vi "Launcher.vi"   [LabVIEW 2020]
uses:
  Controllers/UI Controller/UI Controller/UI Controller.lvclass
  C:/Program Files/National Instruments/LabVIEW 2020/vi.lib/ActorFramework/Actor/Actor.lvclass
  Controllers/UI Controller/Factories/Full Factory/Full Factory.lvclass
  E:/Git/Labview-Projects/Completed projects/Map Editor/Controllers/UI Controller/Factories/UI Factory/UI Factory.lvclass
  Controllers/UI Controller/UI Controller/UI Controller.lvclass/UI Controller.ctl
  <vilib>/ActorFramework/Actor/Actor.lvclass
panel:
  # "NOTICE -- YOU MUST LEAVE THIS NOTICE IN PLACE.\n\nCopyright (c) 2017, LIANG LIU Shawn.Liu.cn@gmail.com\nAll rights reserved.\n\nRedistribution and use in source and binary forms, with or without modification, are permitted provided that the following conditions are met:\n-Redistributions of source code must retain the above copyright notice, this list of conditions and the following disclaimer.\n-Redistributions in binary form must reproduce the above copyright notice, this list of conditions and the following disclaimer in the documentation and/or other materials provided with the distribution.\n-Neither the name of the eLp nor the names of its contributors may be used to endorse or promote products derived from this software without specific prior written permission.\n\nTHIS SOFTWARE IS PROVIDED BY THE COPYRIGHT HOLDERS AND CONTRIBUTORS \"AS IS\" AND ANY EXPRESS OR IMPLIED WARRANTIES, INCLUDING, BUT NOT LIMITED TO, THE IMPLIED WARRANTIES OF MERCHANTABILITY AND FITNESS FOR A PARTICULAR PURPOSE ARE DISCLAIMED. IN NO EVENT SHALL THE COPYRIGHT HOLDER OR CONTRIBUTORS BE LIABLE FOR ANY DIRECT, INDIRECT, INCIDENTAL, SPECIAL, EXEMPLARY, OR CONSEQUENTIAL DAMAGES (INCLUDING, BUT NOT LIMITED TO, PROCUREMENT OF SUBSTITUTE GOODS OR SERVICES; LOSS OF USE, DATA, OR PROFITS; OR BUSINESS INTERRUPTION) HOWEVER CAUSED AND ON ANY THEORY OF LIABILITY, WHETHER IN CONTRACT, STRICT LIABILITY, OR TORT (INCLUDING NEGLIGENCE OR OTHERWISE) ARISING IN ANY WAY OUT OF THE USE OF THIS SOFTWARE, EVEN IF ADVISED OF THE POSSIBILITY OF SUCH DAMAGE."
types:
  T1 = enum32{"invalid app kind", "Development System", "Run Time System", "Student Edition", "Embedded LabVIEW", "Evaluation", "Custom"}
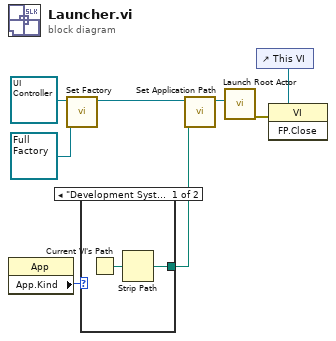
[diagram p0: block diagram]
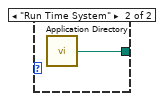
[diagram p2: hidden frame]
diagram:
  n1 = property class="App"() -> ("App.Kind"=w2:T1)  [unwired: 2 in, 2 out]
  n2 = call "Set Factory.vi"("Factory"=refnum<class "Full Factory.lvclass"> refnum ("UI Controller.lvlib:Full Factory.lvclass"), "UI Controller in"=refnum<class "UI Controller.lvclass"> refnum ("UI Controller.lvlib:UI Controller.lvclass")) -> ("UI Controller out"=w7:refnum<class "UI Controller.lvclass">)  [unwired: 9 in]
  n3 = case shown="\"Development System\", Default" w2 {
    tunnel: [w9 w11] -> w1
    frame "Development System", Default {
      n4 = Current VI's Path() -> (path=w10:path)
      n5 = Strip Path(path=w10) -> (stripped path=w9:path)  [unwired: 1 out]
    }
    frame "Run Time System" {
      n6 = call <vilib>:"Application Directory.vi"() -> ("Application Directory"=w11:path)
    }
  }
  n7 = call "Set Application Path.vi"("Application Path"=w1, "UI Controller in"=w7) -> ("UI Controller out"=w3:refnum<class "UI Controller.lvclass">)  [unwired: 9 in]
  n8 = call <vilib>:"Launch Root Actor.vi"("Actor"=w3) -> ("error out"=w5:errorcluster)  [unwired: 9 in, 1 out]
  n9 = control-ref of="This VI"() -> (w4:refnum<vi>)
  n10 = invoke class="VI" method="FP.Close"(reference=w4, error in=w5) -> ()  [unwired: 1 in, 3 out]
